vi "test_MultipleSessionsReserved_CallCloseSessions_SessionsClosed.vi"(8 "error in":errorcluster) -> (0 "error out":errorcluster, 2 "result":string, 3 "pass":bool)   [LabVIEW 2020, in "MeasurementServerTests.lvlib"]
uses:
  MeasurementServerTests.lvlib
  Runtime/APIs/Session Management V1/Session Reservation/Session Reservation.lvclass
  Runtime/APIs/Session Management V1/Session Reservation/Connection.ctl
  Runtime/APIs/Session Management V1/Session Reservation/Connection with Session.ctl
  Helpers/Fake Session Factory/Fake Session Factory.lvclass
  7a2c3fac-9cf0-43a9-826b-68a2a2220f5c.vi
  fcfa9d35-7183-4261-888a-3af72f186d73.vi
  Runtime/APIs/Session Management V1/Session Reservation/Pin Type.ctl
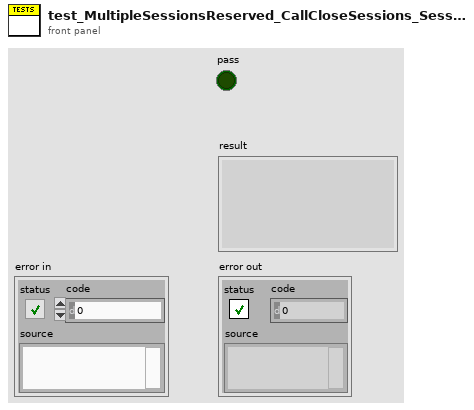
[diagram p1: front panel]
types:
  T1 = typedef "Plug-In SDK Session Management V1 API.lvlib/Session Reservation.lvclass/Pin Type.ctl" = enum16{"DUT and System Pins", "System Pins"}
  T2 = typedef "Plug-In SDK Session Management V1 API.lvlib/Session Reservation.lvclass/Connection with Session.ctl" = cluster{"connection":T3, "session":variant}
  T3 = typedef "Plug-In SDK Session Management V1 API.lvlib/Session Reservation.lvclass/Connection.ctl" = cluster{"pin or relay name":string, "site":i32, "instrument type id":string, "channel":string}
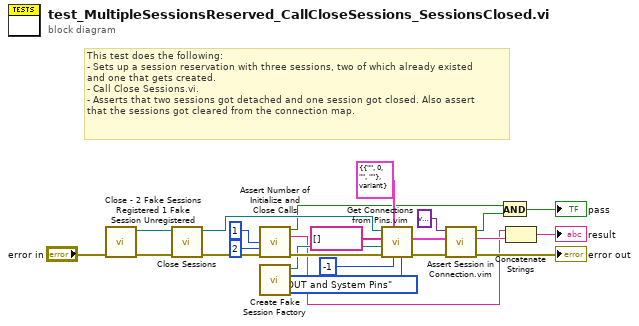
[diagram p0: block diagram]
diagram:
  # "This test does the following:\n- Sets up a session reservation with three sessions, two of which already existed\nand one that gets created.\n- Call Close Sessions.vi.\n- Asserts that two sessions got detached and one session got closed. Also assert \nthat the sessions got cleared from the connection map."
  n1 = call "Close - 2 Fake Sessions Registered 1 Fake Session Unregistered.vi"("error in"="error in") -> ("error out"=w21:errorcluster, "session reservation out"=w20:refnum<class "Session Reservation.lvclass">)  [unwired: 9 in]
  n2 = call "Close Sessions.vi"("error in"=w21, "session reservation in"=w20) -> ("error out"=w19:errorcluster, "session reservation out"=w9:refnum<class "Session Reservation.lvclass">)  [unwired: 8 in]
  n3 = call "Assert Number of Initialize and Close Calls.vi"("expected close-close calls"=u32 1, "expected close-detach calls"=u32 2, "error in"=w19) -> ("pass"=w5:bool, "result"=w2:string, "error out"=w12:errorcluster)  [unwired: 10 in]
  n4 = call "Create Fake Session Factory.vi"() -> ("fake session factory out"=w10:refnum<class "Fake Session Factory.lvclass">)  [unwired: 10 in, 1 out]
  n5 = call "Get Connections from Pins.vim"("pin type"=Pin_Type."DUT and System Pins", "site"=-1, "connection type"=T2 {"connection"={"pin or relay name"="", "site"=0, "instrument type id"="", "channel"=""}, "session"=variant}, "error in"=w12, "session factory"=w10, "pin or relay names"=string[] [], "session reservation in"=w9) -> ("error out"=→"error out":errorcluster, "connections"=w14:T2[])  [unwired: 2 in, 1 out]
  n6 = call "Assert Session in Connection.vim"("actual connections"=w14, "expected session"=variant) -> ("result"=w3:string, "pass"=w7:bool)  [unwired: 8 in]
  n7 = And(x=w5, y=w7) -> (x .and. y?=→"pass":bool)
  n8 = Concatenate Strings(w2, w3) -> (→"result":string)
